vi "Get-file-contents.vi"(8 "error in (no error)":errorcluster, 11 "Reference in":T1) -> (0 "error out":errorcluster, 2 "File contents":string[](array[string]), 3 "Reference out":T1)   [LabVIEW 2013, in "HardwareCharacterization.lvlib" / "HC-ScanParser.lvclass"]
uses:
  HC-ScanParser.lvclass
  Object-reference.ctl
  HC-ScanParser.lvclass/HC-ScanParser.ctl
  Read Scan file path.vi
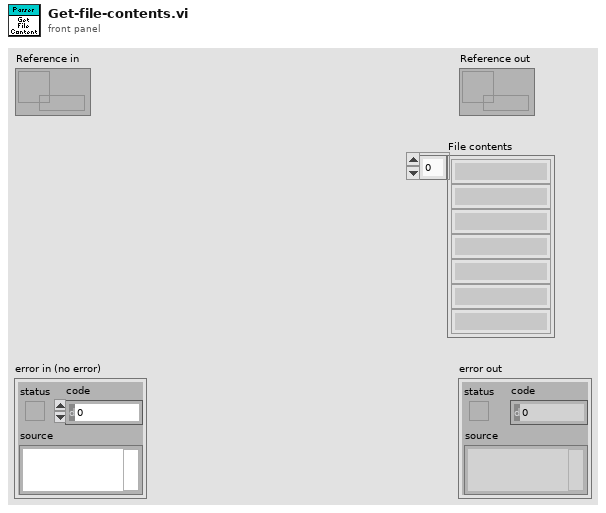
[diagram p1: front panel]
types:
  T1 = typedef "HardwareCharacterization.lvlib/HC-ScanParser.lvclass/Object-reference.ctl" = refnum<data-value>
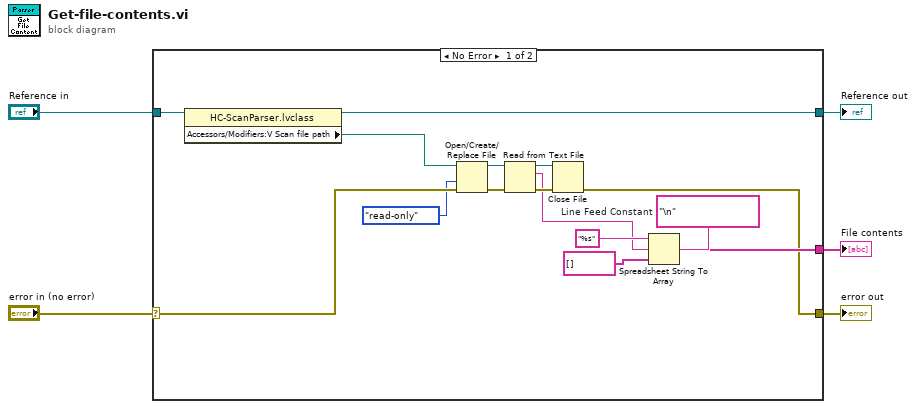
[diagram p0: block diagram]
diagram:
  n1 = case shown="No Error" "error in (no error)" {
    selector: "error in (no error)" -> [w10 w21]
    tunnel: [w6 w21] -> w4
    tunnel: [w16 w22] -> w2
    tunnel: "Reference in" -> [w20 w22]
    tunnel: [w15 _] -> w1
    frame No Error {
      w18 = "\n"  # Line Feed Constant
      n2 = property class="HC-ScanParser.lvclass"(reference=w20) -> (reference out=w16:T1, "Accessors/Modifiers:V Scan file path"=w9:path)  [unwired: 1 in, 1 out]
      n3 = Open/Create/Replace File(file path (use dialog)=w9, error in=w10, access (0:read/write)=enum16{"read/write", "read-only", "write-only"}."read-only") -> (refnum out=w14:refnum<file>, error out=w11:errorcluster)  [unwired: 3 in, 1 out]
      n4 = Read from Text File(file (use dialog)=w14, error in=w11) -> (refnum out=w13:refnum<file>, text=w7:string, error out=w12:errorcluster)  [unwired: 2 in, 1 out]
      n5 = Close File(refnum=w13, error in=w12) -> (error out=w6:errorcluster)  [unwired: 1 out]
      n6 = Spreadsheet String To Array(delimiter (Tab)=w18, format string="%s", spreadsheet string=w7, array type (2D Dbl)=string[] []) -> (array=w15:string[])
    }
    frame Error {
    }
  }
  "error out" <- w4
  "Reference out" <- w2
  "File contents" <- w1
